vi "Parse Pattern String.vi"(9 "Options (Default)":T4, 10 "Encoding Callback":refnum<vi>, 11 "Input":string="{a:foo(bar)b}?") -> (0 "error out":errorcluster, 3 "Part List":T1[](array[typedef]))   [LabVIEW 2020, in "Stream.lvlib" / "URLPattern.lvclass"]
uses:
  URLPattern.lvclass
  Token Type.ctl
  Pattern Part Type.ctl
  Pattern Part Modifier.ctl
  Pattern Part.ctl
  No-op Encoder.vi
  Pattern String Options.ctl
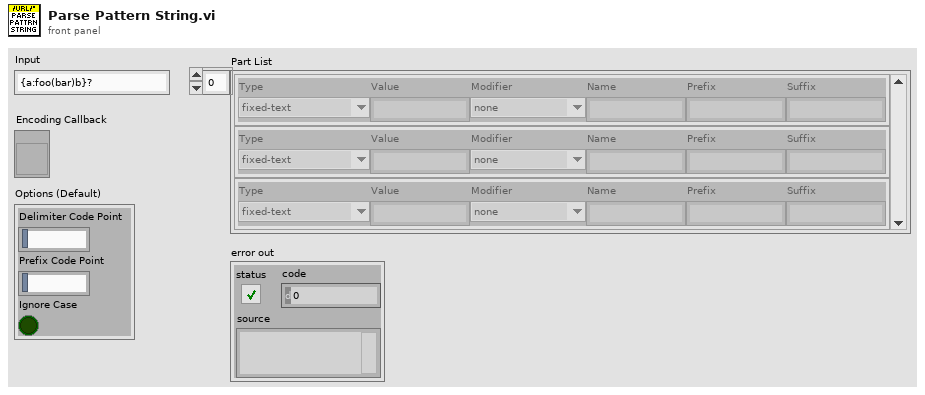
[diagram p1: front panel]
types:
  T1 = typedef "Stream.lvlib/URLPattern.lvclass/Pattern Part.ctl" = cluster{"Type":T2, "Value":string, "Modifier":T3, "Name":string, "Prefix":string, "Suffix":string}
  T2 = typedef "Stream.lvlib/URLPattern.lvclass/Pattern Part Type.ctl" = enum16{"fixed-text", "regexp", "segment-wildcard", "full-wildcard"}
  T3 = typedef "Stream.lvlib/URLPattern.lvclass/Pattern Part Modifier.ctl" = enum16{"none", "optional", "zero-or-more", "one-or-more"}
  T4 = typedef "Stream.lvlib/URLPattern.lvclass/Pattern String Options.ctl" = cluster{"Delimiter Code Point":string, "Prefix Code Point":string, "Ignore Case":bool}
  T5 = typedef "Stream.lvlib/URLPattern.lvclass/Pattern Parser.ctl" = cluster{"Token List":T6[], "Encoding Callback":refnum<vi>, "Segment Wildcard Regexp":string, "Part List":T1[], "Pending Fixed Value":string, "Index":i32, "Next Numeric Name":i32, "Token Length":i32}
  T6 = typedef "Stream.lvlib/URLPattern.lvclass/Token.ctl" = cluster{"Type":T7, "Index":i32, "Value":string}
  T7 = typedef "Stream.lvlib/URLPattern.lvclass/Token Type.ctl" = enum16{"invalid-char", "open", "close", "regexp", "name", "char", "escaped-char", "other-modifier", "asterisk", "end"}
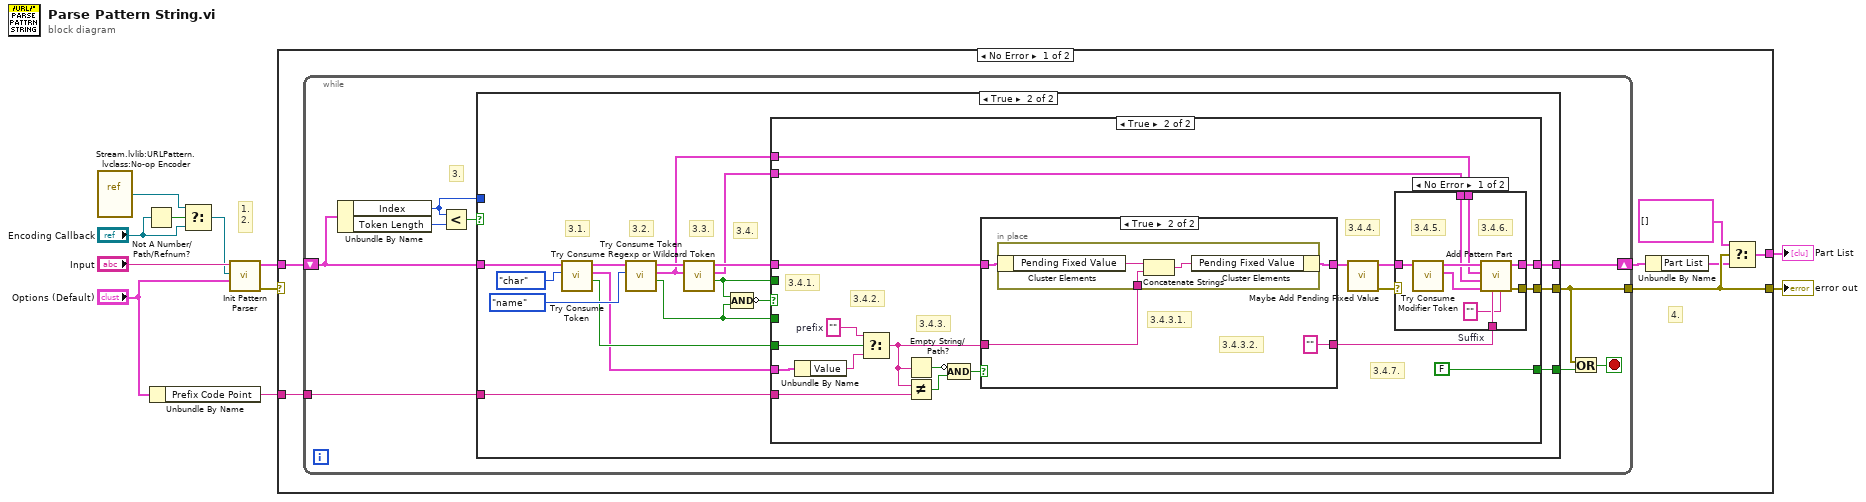
[diagram p0: block diagram]
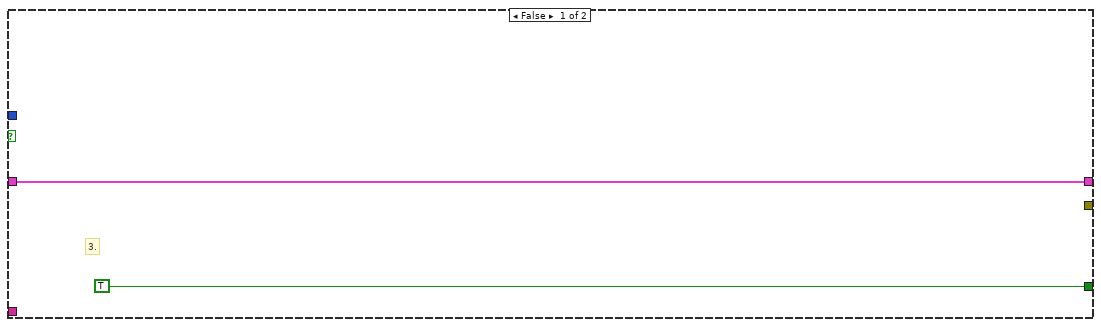
[diagram p2: hidden frame]
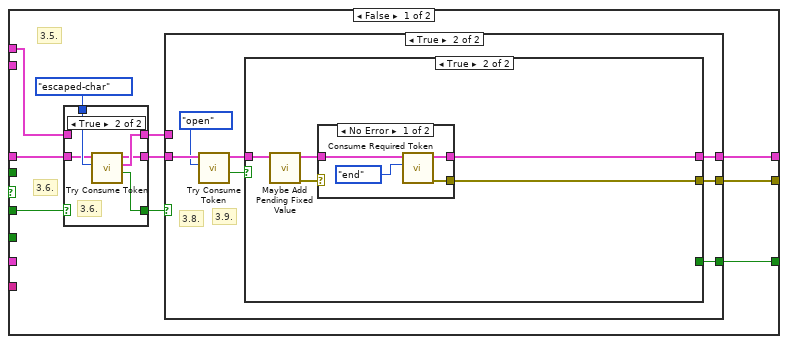
[diagram p3: hidden frame]
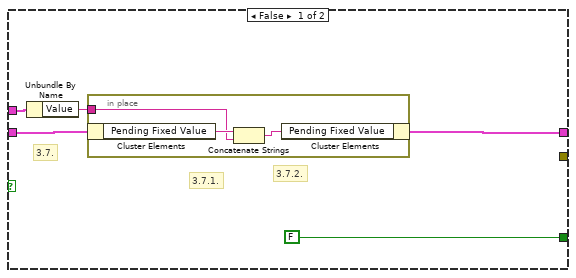
[diagram p4: hidden frame]
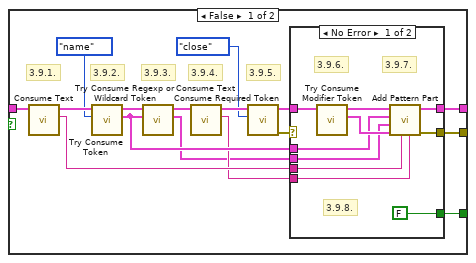
[diagram p5: hidden frame]
diagram:
  # "1.\n2."
  n1 = vi-ref "Stream.lvlib:URLPattern.lvclass:No-op Encoder.vi"() -> (w2:refnum<vi>)
  n2 = Not A Number/Path/Refnum?(number/path/refnum="Encoding Callback") -> (NaN/Path/Refnum?=w4:bool)
  n3 = Unbundle By Name("Options (Default)") -> ("Prefix Code Point"=w7:string)
  n4 = Select(t=w2, s=w4, f="Encoding Callback") -> (s? t:f=w1:refnum<vi>)
  n5 = call "Init Pattern Parser.vi"("Options"="Options (Default)", "Encoding Callback"=w1, "Input"="Input") -> ("error out"=w9:errorcluster, "Pattern Parser"=w11:T5)  [unwired: 7 in]
  n6 = case shown="No Error" w9 {
    selector: w9 -> [_ w158]
    tunnel: w11 -> [w12 _]
    tunnel: w7 -> [w17 _]
    tunnel: [w18 w158] -> w6
    tunnel: [w14 _] -> w5
    frame No Error {
      # "4."
      n7 = while {
        shift-right: [w22] -> w16
        shift-left: w12 -> [w24]
        tunnel: w17 -> [w21]
        tunnel: [w19] -> w18
        stop <- w20 stop-if-true
        # "3."
        n8 = Unbundle By Name(w24) -> ("Index"=w25:i32, "Token Length"=w27:i32)
        n9 = Less?(x=w25, y=w27) -> (x < y?=w26:bool)
        n10 = case shown="True" w26 {
          tunnel: w25 -> [_ _]
          tunnel: w24 -> [w28 w46]
          tunnel: [TRUE w32] -> w23
          tunnel: [w28 w34] -> w22
          tunnel: w21 -> [_ w35]
          tunnel: [_ w33] -> w19
          frame False {
            # "3."
          }
          frame True {
            # "3.4."
            # "3.3."
            # "3.2."
            # "3.1."
            n11 = call "Try Consume Token.vi"("Type"=Token_Type."char", "Pattern Parser In"=w46) -> ("Null?"=w39:bool, "Token"=w36:T6, "Pattern Parser"=w44:T5)  [unwired: 7 in]
            n12 = call "Try Consume Token.vi"("Type"=Token_Type."name", "Pattern Parser In"=w44) -> ("Null?"=w31:bool, "Token"=w38:T6, "Pattern Parser"=w42:T5)  [unwired: 7 in]
            n13 = call "Try Consume Regexp or Wildcard Token.vi"("Name Token"=w38, "Pattern Parser In"=w42) -> ("Null?"=w30:bool, "Token"=w37:T6, "Pattern Parser"=w41:T5)  [unwired: 7 in]
            n14 = Compound Arithmetic op=AND(w30, w31) -> (invert w40:bool)
            n15 = case shown="True" w40 {
              tunnel: w41 -> [w55 w129]
              tunnel: w39 -> [_ w137]
              tunnel: w38 -> [w53 w124]
              tunnel: w37 -> [_ w123]
              tunnel: w36 -> [_ w136]
              tunnel: w35 -> [_ w133]
              tunnel: [w49 w122] -> w34
              tunnel: [w47 w121] -> w33
              tunnel: [w48 FALSE] -> w32
              tunnel: w31 -> [w56 _]
              tunnel: w30 -> [_ _]
              frame False {
                # "3.6."
                # "3.5."
                n16 = case shown="True" w56 {
                  selector: w56 -> [w111 _]
                  tunnel: w55 -> [w112 w117]
                  tunnel: Token_Type."escaped-char" ("Type") -> [_ w118]
                  tunnel: w53 -> [w113 _]
                  tunnel: [w113 w116] -> w50
                  tunnel: [w112 w115] -> w51
                  tunnel: [w111 w114] -> w52
                  frame False {
                  }
                  frame True {
                    # "3.6."
                    n17 = call "Try Consume Token.vi"("Type"=w118, "Pattern Parser In"=w117) -> ("Null?"=w114:bool, "Token"=w116:T6, "Pattern Parser"=w115:T5)  [unwired: 7 in]
                  }
                }
                n18 = case shown="True" w52 {
                  tunnel: w51 -> [w60 w71]
                  tunnel: w50 -> [w61 _]
                  tunnel: [w58 w67] -> w49
                  tunnel: [FALSE w65] -> w48
                  tunnel: [_ w66] -> w47
                  frame False {
                    # "3.7.2."
                    # "3.7.1."
                    # "3.7."
                    n19 = Unbundle By Name(w61) -> ("Value"=w59:string)
                    n20 = in-place {
                      in-place-border: w59 -> [w62]
                      n21 = in-place-cluster #1(w60) -> ("Pending Fixed Value"=w64:string)
                      n22 = Concatenate Strings(w64, w62) -> (w63:string)
                      n23 = in-place-cluster #1("Pending Fixed Value"=w63) -> (w58:T5)
                    }
                  }
                  frame True {
                    # "3.9."
                    # "3.8."
                    n24 = call "Try Consume Token.vi"("Type"=Token_Type."open", "Pattern Parser In"=w71) -> ("Null?"=w69:bool, "Pattern Parser"=w68:T5)  [unwired: 7 in, 1 out]
                    n25 = case shown="True" w69 {
                      tunnel: w68 -> [w87 w104]
                      tunnel: [w78 w101] -> w67
                      tunnel: [w77 w102] -> w66
                      tunnel: [w72 _] -> w65
                      frame False {
                        # "3.9.5."
                        # "3.9.4."
                        # "3.9.3."
                        # "3.9.2."
                        # "3.9.1."
                        n26 = call "Consume Text.vi"("Pattern Parser In"=w87) -> ("Result"=w75:string, "Pattern Parser"=w86:T5)  [unwired: 9 in]
                        n27 = call "Try Consume Token.vi"("Type"=Token_Type."name", "Pattern Parser In"=w86) -> ("Token"=w76:T6, "Pattern Parser"=w84:T5)  [unwired: 7 in, 1 out]
                        n28 = call "Try Consume Regexp or Wildcard Token.vi"("Name Token"=w76, "Pattern Parser In"=w84) -> ("Token"=w73:T6, "Pattern Parser"=w83:T5)  [unwired: 7 in, 1 out]
                        n29 = call "Consume Text.vi"("Pattern Parser In"=w83) -> ("Result"=w74:string, "Pattern Parser"=w82:T5)  [unwired: 9 in]
                        n30 = call "Consume Required Token.vi"("Type"=Token_Type."close", "Pattern Parser In"=w82) -> ("error out"=w80:errorcluster, "Pattern Parser"=w79:T5)  [unwired: 7 in, 1 out]
                        n31 = case shown="No Error" w80 {
                          selector: w80 -> [_ w99]
                          tunnel: w79 -> [w97 w98]
                          tunnel: [w89 w98] -> w78
                          tunnel: [w90 w99] -> w77
                          tunnel: w76 -> [w94 _]
                          tunnel: w75 -> [w93 _]
                          tunnel: w74 -> [w92 _]
                          tunnel: w73 -> [w91 _]
                          tunnel: [FALSE _] -> w72
                          frame No Error {
                            # "3.9.8."
                            # "3.9.7."
                            # "3.9.6."
                            n32 = call "Try Consume Modifier Token.vi"("Pattern Parser In"=w97) -> ("Token"=w95:T6, "Pattern Parser"=w96:T5)  [unwired: 8 in, 1 out]
                            n33 = call "Add Pattern Part.vi"("Suffix"=w92, "Prefix"=w93, "Modifier Token"=w95, "Regexp or Wildcard Token"=w91, "Name Token"=w94, "Pattern Parser In"=w96) -> ("error out"=w90:errorcluster, "Pattern Parser"=w89:T5)  [unwired: 4 in]
                          }
                          frame Error {
                          }
                        }
                      }
                      frame True {
                        n34 = call "Maybe Add Pending Fixed Value.vi"("Pattern Parser In"=w104) -> ("error out"=w100:errorcluster, "Pattern Parser"=w103:T5)  [unwired: 9 in]
                        n35 = case shown="No Error" w100 {
                          selector: w100 -> [_ w110]
                          tunnel: w103 -> [w108 w109]
                          tunnel: [w106 w110] -> w102
                          tunnel: [w105 w109] -> w101
                          frame No Error {
                            n36 = call "Consume Required Token.vi"("Type"=Token_Type."end", "Pattern Parser In"=w108) -> ("error out"=w106:errorcluster, "Pattern Parser"=w105:T5)  [unwired: 7 in, 1 out]
                          }
                          frame Error {
                          }
                        }
                      }
                    }
                  }
                }
              }
              frame True {
                w134 = ""  # prefix
                # "3.4.7."
                # "3.4.4."
                # "3.4.3."
                # "3.4.2."
                # "3.4.1."
                n37 = Unbundle By Name(w136) -> ("Value"=w135:string)
                n38 = Select(t=w134, s=w137, f=w135) -> (s? t:f=w128:string)
                n39 = Empty String/Path?(string/path=w128) -> (empty?=w132:bool)
                n40 = Not Equal?(x=w128, y=w133) -> (x != y?=w131:bool)
                n41 = Compound Arithmetic op=AND(invert w132, w131) -> (w130:bool)
                n42 = case shown="True" w130 {
                  tunnel: w129 -> [w150 w154]
                  tunnel: w128 -> [w149 w153]
                  tunnel: [w150 w152] -> w127
                  tunnel: [w149 "" ("Value")] -> w125
                  frame False {
                  }
                  frame True {
                    # "3.4.3.1."
                    # "3.4.3.2."
                    n43 = in-place {
                      in-place-border: w153 -> [w156]
                      n44 = in-place-cluster #2(w154) -> ("Pending Fixed Value"=w157:string)
                      n45 = Concatenate Strings(w157, w156) -> (w155:string)
                      n46 = in-place-cluster #2("Pending Fixed Value"=w155) -> (w152:T5)
                    }
                  }
                }
                n47 = call "Maybe Add Pending Fixed Value.vi"("Pattern Parser In"=w127) -> ("error out"=w119:errorcluster, "Pattern Parser"=w126:T5)  [unwired: 9 in]
                n48 = case shown="No Error" w119 {
                  selector: w119 -> [_ w148]
                  tunnel: w126 -> [w146 w147]
                  tunnel: w125 -> [w143 _]
                  tunnel: w124 -> [w142 _]
                  tunnel: w123 -> [w141 _]
                  tunnel: [w139 w147] -> w122
                  tunnel: [w138 w148] -> w121
                  frame No Error {
                    w140 = ""  # Suffix
                    # "3.4.6."
                    # "3.4.5."
                    n49 = call "Try Consume Modifier Token.vi"("Pattern Parser In"=w146) -> ("Token"=w144:T6, "Pattern Parser"=w145:T5)  [unwired: 8 in, 1 out]
                    n50 = call "Add Pattern Part.vi"("Suffix"=w140, "Prefix"=w143, "Modifier Token"=w144, "Regexp or Wildcard Token"=w141, "Name Token"=w142, "Pattern Parser In"=w145) -> ("error out"=w138:errorcluster, "Pattern Parser"=w139:T5)  [unwired: 4 in]
                  }
                  frame Error {
                  }
                }
              }
            }
          }
        }
        n51 = Or(x=w19, y=w23) -> (x .or. y?=w20:bool)
      }
      n52 = Unbundle By Name(w16) -> ("Part List"=w15:T1[])
      n53 = Select(t=T1[] [], s=w18, f=w15) -> (s? t:f=w14:T1[])
    }
    frame Error {
    }
  }
  "error out" <- w6
  "Part List" <- w5
